vi "send inital pos data.vi"(8 "error in (no error)":errorcluster) -> (0 "error out":errorcluster)   [LabVIEW 2014]
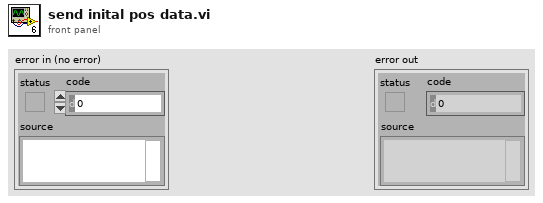
[diagram p1: front panel]
types:
  T1 = typedef "WPI_SerialPortRef.ctl" = cluster{"DevStatus":errorcluster, "Serial Port Name":refnum<visa-resource-name>}
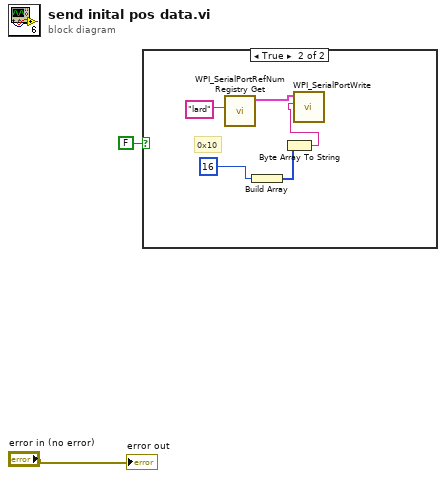
[diagram p0: block diagram]
diagram:
  n1 = case shown="True" FALSE {
    frame False {
    }
    frame True {
      # "0x10"
      n2 = call <vilib>:"WPI_SerialPortRefNum Registry Get.vi"("refnum name"="lard") -> ("SerialPortRef"=w6:T1)  [unwired: 9 in, 1 out]
      n3 = Build Array(u8 16) -> (w3:u8[])
      n4 = Byte Array To String(unsigned byte array=w3) -> (string=w5:string)
      n5 = call <vilib>:"WPI_SerialPortWrite.vi"("Buffer"=w5, "SerialPortRef"=w6) -> ()  [unwired: 7 in, 3 out]
    }
  }
  "error out" <- "error in (no error)"
